vi "TinyTCP Control.vi"() -> ()   [LabVIEW 2020]
uses:
  TCP Comms/Instance.ctl
  TCP Comms/Ref Data.ctl
  TCP Comms/State.ctl
  TCP Comms/TinyTCP.lvlib
panel:
  in  "TinyTCP":T1
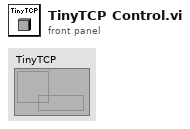
[diagram p1: front panel]
types:
  T1 = typedef "TinyTCP.lvlib/Instance.ctl" = refnum<data-value>
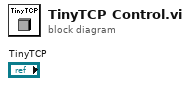
[diagram p0: block diagram]
diagram:
